vi "Merge Data.vi"(8 "error in":errorcluster, 10 "Analyzed":refnum<class "Instrument.lvclass">, 11 "Acquired":refnum<class "CRDS.lvclass">) -> (0 "error out":errorcluster, 3 "CRDS out":refnum<class "CRDS.lvclass">)   [LabVIEW 2015, in "CRDS Lib.lvlib" / "CRDS.lvclass"]
doc: "The VI Merge Data is used strictly here to merge the serial data with the rest of the data. THIS VI WILL BE NO LONGER NECESSARY WHEN ISSUES RELATING TO RT EXE ARE FIXED!!"
uses:
  CRDS.lvclass
  Instrument/Instrument.lvclass
  Data/Main/CRDS Data.lvclass
  Instrument/Instrument.lvclass/Instrument.ctl
  Cell/CRDS Cell.lvclass/CRDS Cell.ctl
  Data/Cell/CRDS Cell Data.lvclass/CRDS Cell Data.ctl
  Cell/Read Data.vi
  Data/Cell/Read extParam.vi
  Data/Cell/Write extParam.vi
  Cell/Write Data.vi
  Instrument/Read Data.vi
  Instrument/Write Data.vi
  Read Cells.vi
  Cell/Read corr tau0.vi
  Cell/Read tau_0.vi
  Cell/Write corr tau0.vi
  Cell/Write tau_0.vi
  Write Cells.vi
  Cell/CRDS Cell.lvclass
  Data/Data.lvclass
  Data/Cell/CRDS Cell Data.lvclass
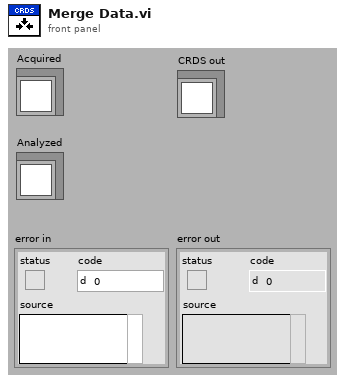
[diagram p1: front panel]
types:
  T1 = typedef "extparam.ctl" = cluster{"Tau":sgl, "Tau0cor":sgl, "ext":sgl, "extCorr":sgl, "stdevTau":sgl, "eTau":sgl, "taucorr":sgl, "Tau0":sgl, "max":sgl}
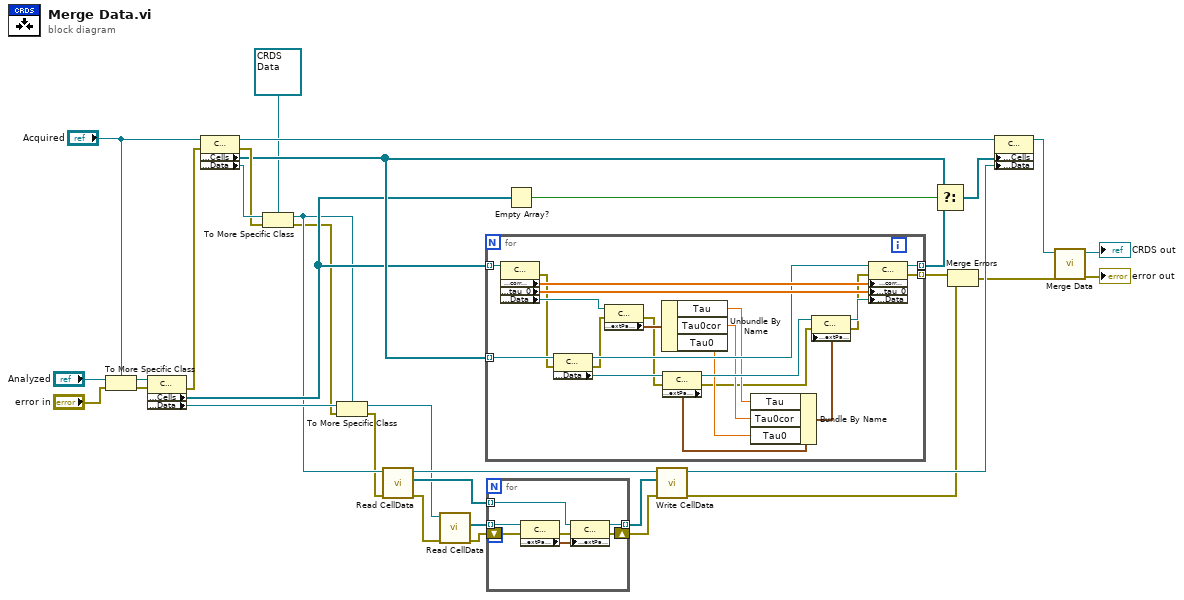
[diagram p0: block diagram]
diagram:
  n1 = To More Specific Class(target class="Acquired", reference="Analyzed", error in="error in") -> (specific class reference=w32:refnum<class "CRDS.lvclass">, error out=w6:errorcluster)
  n2 = property class="CRDS"(reference=w32, error in=w6) -> (error out=w5:errorcluster, "Data Access:Cells"=w13:refnum<class "CRDS Cell.lvclass">[], "Accessors:Data"=w12:refnum<class "Data.lvclass">)  [unwired: 1 out]
  n3 = property class="CRDS"(reference="Acquired", error in=w5) -> (reference out=w27:refnum<class "CRDS.lvclass">, error out=w29:errorcluster, "Data Access:Cells"=w28:refnum<class "CRDS Cell.lvclass">[], "Accessors:Data"=w30:refnum<class "Data.lvclass">)
  n4 = To More Specific Class(target class=refnum<class "CRDS Data.lvclass"> refnum ("Data"), reference=w30, error in=w29) -> (specific class reference=w4:refnum<class "CRDS Data.lvclass">, error out=w3:errorcluster)
  n5 = To More Specific Class(target class=w4, reference=w12, error in=w3) -> (specific class reference=w11:refnum<class "CRDS Data.lvclass">, error out=w2:errorcluster)
  n6 = call "Read CellData.vi"("error in"=w2, "CRDS Data in"=w4) -> ("error out"=w19:errorcluster, "CellData"=w17:refnum<class "CRDS Cell Data.lvclass">[], "CRDS Data out"=w20:refnum<class "CRDS Data.lvclass">)  [unwired: 7 in]
  n7 = call "Read CellData.vi"("error in"=w19, "CRDS Data in"=w11) -> ("error out"=w22:errorcluster, "CellData"=w18:refnum<class "CRDS Cell Data.lvclass">[])  [unwired: 7 in, 1 out]
  n8 = for {
    tunnel: w13 -> [w56] mode=indexing
    tunnel: w28 -> [w51] mode=indexing
    tunnel: [w53] -> w23 mode=indexing
    tunnel: [w41] -> w16 mode=indexing
    n9 = property class="CRDS Cell"(reference=w56) -> (error out=w40:errorcluster, "Accessors:corr tau0"=w55:dbl[], "Accessors:tau_0"=w54:dbl[], "Accessors:Data"=w52:refnum<class "CRDS Cell Data.lvclass">)  [unwired: 1 in, 1 out]
    n10 = property class="CRDS Cell"(reference=w51, error in=w40) -> (reference out=w50:refnum<class "CRDS Cell.lvclass">, error out=w39:errorcluster, "Accessors:Data"=w49:refnum<class "CRDS Cell Data.lvclass">)
    n11 = property class="CRDS Cell"(reference=w52, error in=w39) -> (error out=w38:errorcluster, "Data Access:extParam"=w46:T1)  [unwired: 1 out]
    n12 = Unbundle By Name(w46) -> ("Tau"=w37:sgl, "Tau0cor"=w45:sgl, "Tau0"=w44:sgl)
    n13 = property class="CRDS Cell"(reference=w49, error in=w38) -> (reference out=w47:refnum<class "CRDS Cell Data.lvclass">, error out=w36:errorcluster, "Data Access:extParam"=w48:T1)
    n14 = Bundle By Name(cluster=w48, "Tau"=w37, "Tau0cor"=w45, "Tau0"=w44) -> (w43:T1)
    n15 = property class="CRDS Cell"(reference=w47, error in=w36, "Data Access:extParam"=w43) -> (reference out=w42:refnum<class "CRDS Cell Data.lvclass">, error out=w35:errorcluster)
    n16 = property class="CRDS Cell"(reference=w50, error in=w35, "Accessors:corr tau0"=w55, "Accessors:tau_0"=w54, "Accessors:Data"=w42) -> (reference out=w53:refnum<class "CRDS Cell.lvclass">, error out=w41:errorcluster)
  }
  n17 = for "Insert extinction data" {
    tunnel: w18 -> [w63] mode=indexing
    tunnel: w17 -> [w59] mode=indexing
    tunnel: [w57] -> w21 mode=indexing
    shift-right: [w58] -> w1
    shift-left: w22 -> [w62]
    n18 = property class="CRDS Cell"(reference=w63, error in=w62) -> (error out=w60:errorcluster, "Data Access:extParam"=w61:T1)  [unwired: 1 out]
    n19 = property class="CRDS Cell"(reference=w59, error in=w60, "Data Access:extParam"=w61) -> (reference out=w57:refnum<class "CRDS Cell Data.lvclass">, error out=w58:errorcluster)
  }
  n20 = Empty Array?(array=w13) -> (empty?=w14:bool)
  n21 = call "Write CellData.vi"("error in"=w1, "CellData"=w21, "CRDS Data in"=w20) -> ("error out"=w15:errorcluster, "CRDS Data out"=w25:refnum<class "CRDS Data.lvclass">)  [unwired: 7 in]
  n22 = Select(t=w28, s=w14, f=w23) -> (s? t:f=w26:refnum<class "CRDS Cell.lvclass">[])
  n23 = Merge Errors(w16, w15) -> (w8:errorcluster)
  n24 = property class="CRDS"(reference=w27, "Data Access:Cells"=w26, "Accessors:Data"=w25) -> (reference out=w10:refnum<class "CRDS.lvclass">)  [unwired: 1 in, 1 out]
  n25 = call-parent "Merge Data.vi"("error in"=w8, "Acquired"=w10) -> ("error out"=→"error out":errorcluster, "Instrument out"=→"CRDS out":refnum<class "CRDS.lvclass">)  [unwired: 8 in]
